vi "main.vi"() -> ()   [LabVIEW 2020, in "Resonance Curve.lvclass"]
uses:
  Resonance Curve.lvclass
  Keysight 33500B/Keysight 33511B.lvclass
  C:/Users/jhko7/Desktop/LabVIEW Programs/AFM Control/Function Generator/Function Generator.lvclass
  SR 830 & NI USB7855R/SR 830 & NI USB7855R.lvclass
  C:/Users/jhko7/Desktop/LabVIEW Programs/AFM Control/Lock-In Amplifier/Lock-In Amplifier.lvclass
  Resonance Curve Data/Resonance Curve Data.lvclass
  Resonance Curve.lvclass/Resonance Curve.ctl
panel:
  in  "Stop All":bool
  in  "Tab Control":enum32{"Measurement", "Setup"}(tab)
  in  "Stop acquisition":bool
  in  "Save Resonance Curve":bool
  out "Current amplitude":dbl
  out "Resonance curve plot":cluster{dbl[], dbl[]}[](graph)
  in  "Start Measurement":bool
  out "Current phase":dbl
  in  "error in":errorcluster
  in  "Wait time (ms)":u32=100
  in  "Driving amplitude (V rms)":dbl=0.001
  in  "Center frequency":dbl=40.0
  out "Coarse range end":dbl=32796.3
  out "Fine range end":dbl=32761.3
  out "Fine range start":dbl=32751.3
  out "Coarse range start":dbl=32716.3
  in  "Apply \nMeasurement Spec":bool
  in  "Coarse range":dbl=40.0
  in  "Fine range":dbl=5.0
  in  "Coarse increment":dbl=1.0
  in  "Fine increment":dbl=0.5
  in  "SR 830 & NI USB7855R Lock-In Amplifier":refnum<class "SR 830 & NI USB7855R.lvclass">
  in  "Keysight 33511B Waveform Generator":refnum<class "Keysight 33511B.lvclass">
  # "Measurement Frequency Select"
  # "Frequency Sweep"
  # "Resonance Curve"
  # "Range"
  # "delta"
  # "Fine"
  # "Coarse"
  # "Full Range"
  # "Fine Range"
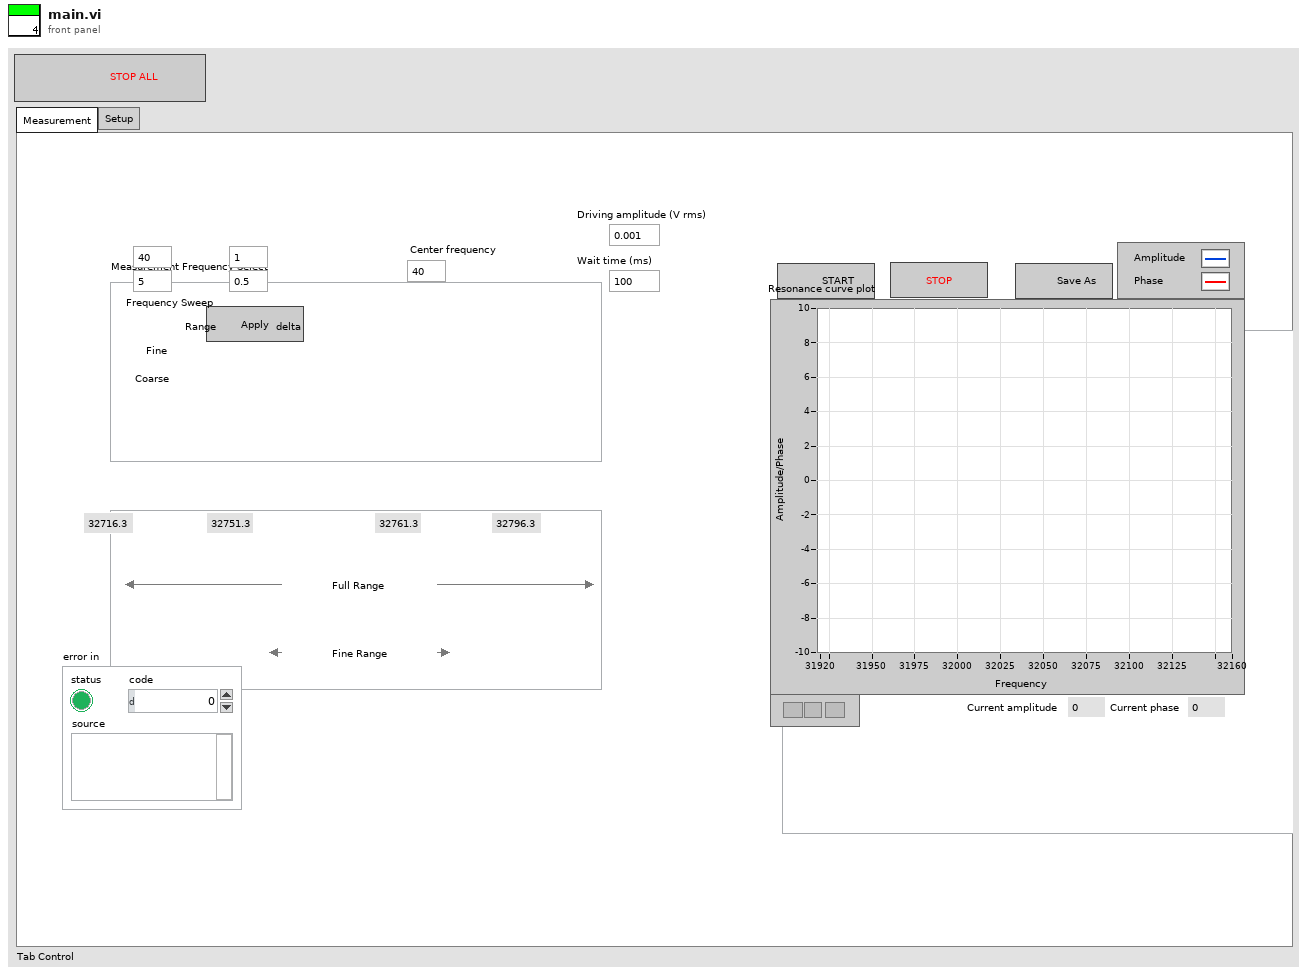
[diagram p1: front panel]
types:
  T1 = cluster{"Frequency (Hz)":dbl[], "Amplitude(V) / Phase (rad)":dbl[]}[]
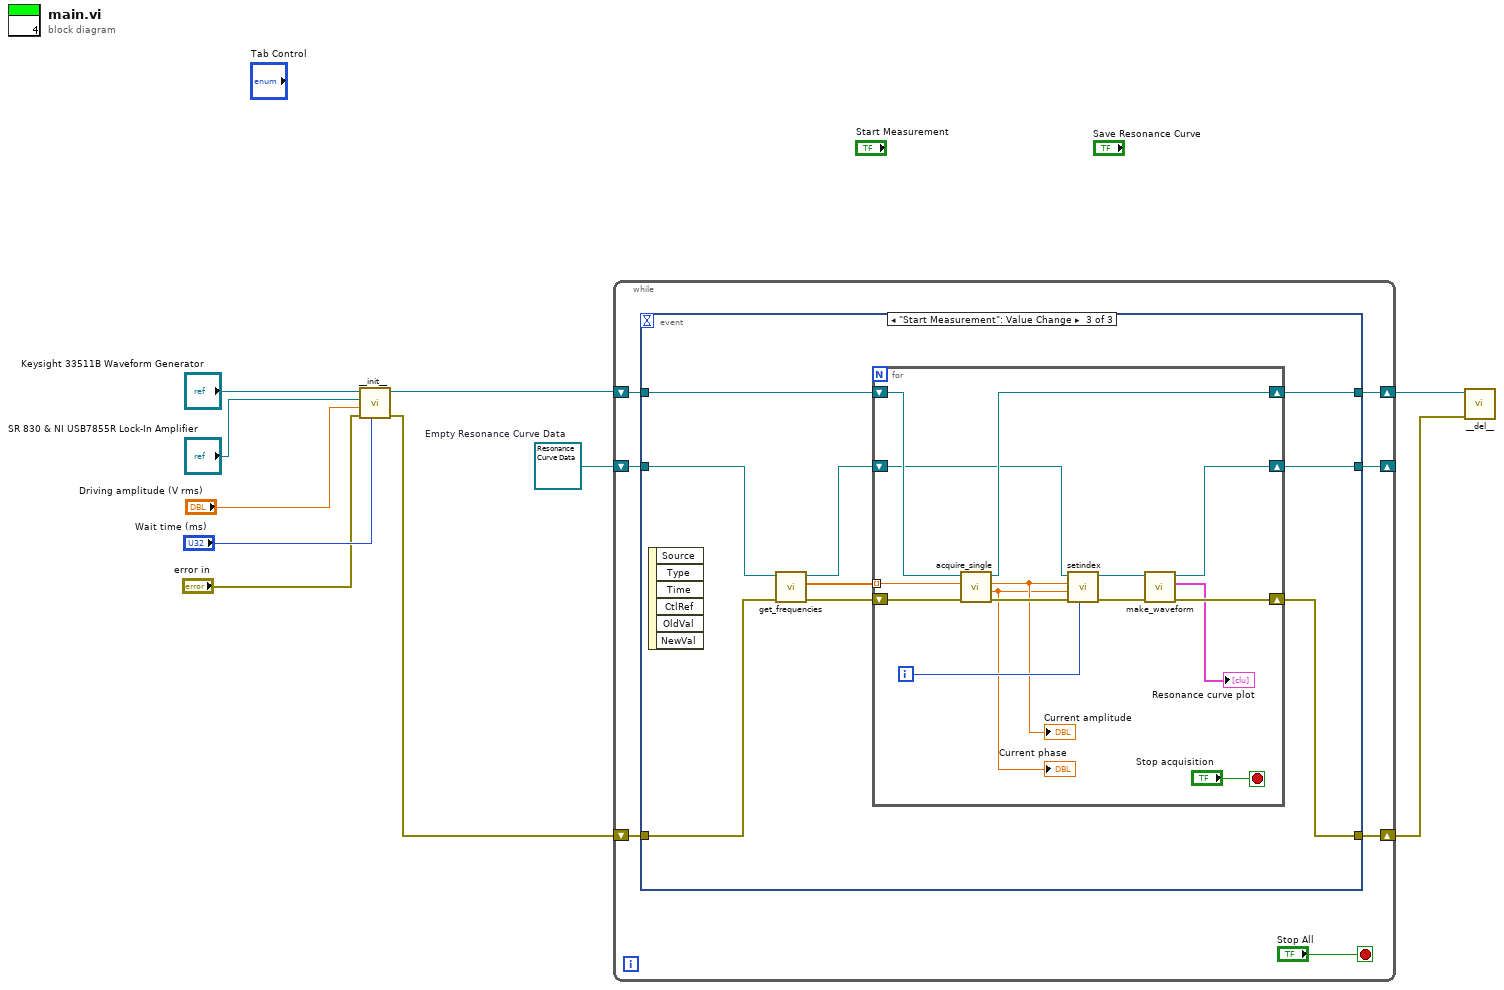
[diagram p0: block diagram]
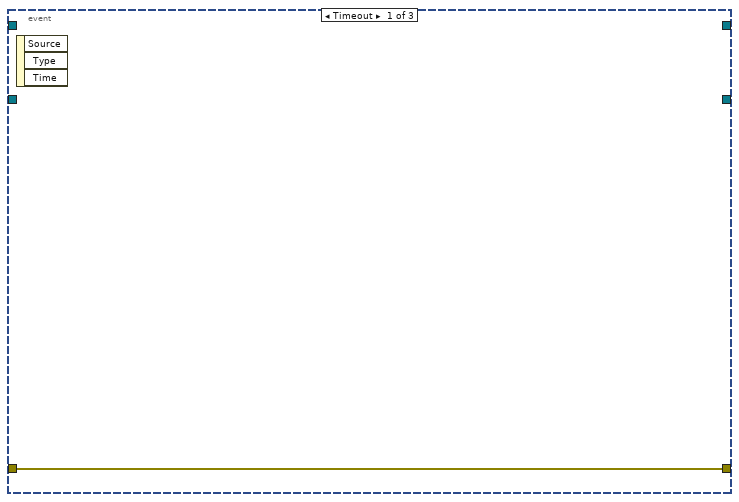
[diagram p2: hidden frame]
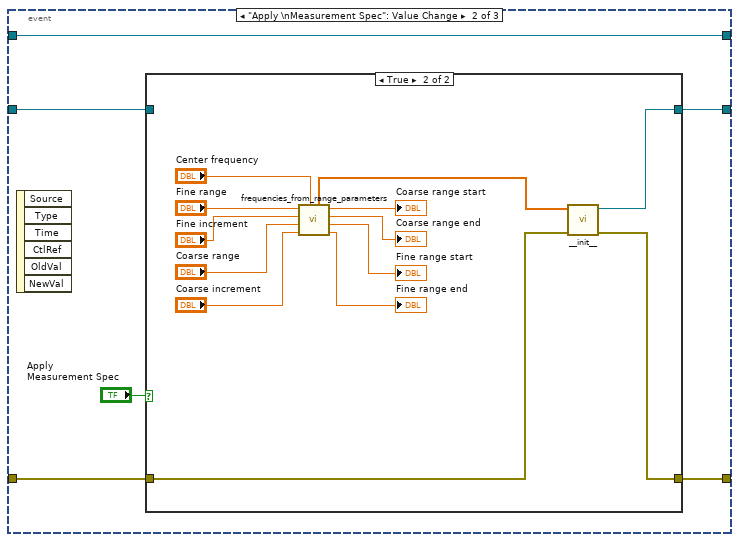
[diagram p3: hidden frame]
diagram:
  w3 = refnum<class "Resonance Curve Data.lvclass"> refnum  # Empty Resonance Curve Data
  n1 = call "__init__.vi"("Wait Time (ms)"="Wait time (ms)", "error in"="error in", "Driving Amplitude (V rms)"="Driving amplitude (V rms)", "Lock-In Amplifier"="SR 830 & NI USB7855R Lock-In Amplifier", "Function Generator"="Keysight 33511B Waveform Generator") -> ("error out"=w4:errorcluster, "Initialized Resonance Curve Measurement"=w5:refnum<class "Resonance Curve.lvclass">)  [unwired: 5 in]
  n2 = while {
    shift-right: [w14] -> w2
    shift-left: w5 -> [w17]
    shift-right: [w13] -> w1
    shift-left: w4 -> [w12]
    shift-right: [w15] -> _
    shift-left: w3 -> [w16]
    stop <- "Stop All" stop-if-true
    n3 = event shown="[2] \"Start Measurement\": Value Change" {
      selector: _ -> [_ _ _]
      dyn-events: _ -> [_ _ _]
      timeout: _ -> [_ _ _]
      tunnel: w12 -> [w18 w23 w47]
      tunnel: [w18 w22 w40] -> w13
      tunnel: w17 -> [_ w24 w42]
      tunnel: w16 -> [_ w20 w48]
      tunnel: [_ w21 w43] -> w15
      tunnel: [_ w24 w41] -> w14
      event Timeout {
        n4 = event-data() -> ()  [unwired: 1 in, 3 out]
      }
      event "Apply \nMeasurement Spec": Value Change {
        n5 = event-data() -> ()  [unwired: 1 in, 6 out]
        n6 = case shown="True" "Apply \nMeasurement Spec" {
          tunnel: w23 -> [w26 w29]
          tunnel: [w26 w28] -> w22
          tunnel: [w25 w27] -> w21
          tunnel: w20 -> [w25 _]
          frame False {
          }
          frame True {
            n7 = call "frequencies_from_range_parameters.vi"("Center frequency (Hz)"="Center frequency", "Fine increment (Hz)"="Coarse increment", "Fine range width (Hz)"="Coarse range", "Coarse increment (Hz)"="Fine increment", "Coarse range width (Hz)"="Fine range") -> ("Fine range end (Hz)"=→"Fine range end":dbl, "Fine range start (Hz)"=→"Fine range start":dbl, "Coarse range end (Hz)"=→"Coarse range end":dbl, "Coarse range start (Hz)"=→"Coarse range start":dbl, "Measurement frequencies (Hz)"=w30:dbl[])  [unwired: 2 in]
            n8 = call "__init__.vi"("error in (no error)"=w29, "Frequencies"=w30) -> ("error out"=w28:errorcluster, "Resonance Curve Data out"=w27:refnum<class "Resonance Curve Data.lvclass">)  [unwired: 8 in]
          }
        }
      }
      event "Start Measurement": Value Change {
        n9 = event-data() -> ()  [unwired: 1 in, 6 out]
        n10 = call "get_frequencies.vi"("error in"=w47, "Resonance Curve Data in"=w48) -> ("error out"=w46:errorcluster, "Frequencies (Hz)"=w45:dbl[], "Resonance Curve Data out"=w44:refnum<class "Resonance Curve Data.lvclass">)  [unwired: 7 in]
        n11 = for {
          tunnel: w45 -> [w63] mode=indexing
          shift-right: [w52] -> w43
          shift-left: w44 -> [w57]
          shift-right: [w60] -> w41
          shift-left: w42 -> [w61]
          shift-right: [w51] -> w40
          shift-left: w46 -> [w62]
          i -> [w58]
          stop <- "Stop acquisition" stop-if-true
          n12 = call-dynamic "acquire_single.vi"("error in (no error)"=w62, "Frequency (Hz)"=w63, "Resonance Curve in"=w61) -> ("error out"=w59:errorcluster, "Phase (rad)"=w55:dbl, "Amplitude (V rms)"=w56:dbl, "Resonance Curve out"=w60:refnum<class "Resonance Curve.lvclass">)  [unwired: 5 in]
          "Current amplitude" <- w56
          "Current phase" <- w55
          n13 = call "setindex.vi"("Index"=w58, "error in"=w59, "Phase (rad)"=w55, "Amplitude (V)"=w56, "Resonance Curve Data in"=w57) -> ("error out"=w53:errorcluster, "Resonance Curve Data out"=w54:refnum<class "Resonance Curve Data.lvclass">)  [unwired: 5 in]
          n14 = call "make_waveform.vi"("error in"=w53, "Resonance Curve Data in"=w54) -> ("error out"=w51:errorcluster, "2D waveform out"=→"Resonance curve plot":T1, "Resonance Curve Data out"=w52:refnum<class "Resonance Curve Data.lvclass">)  [unwired: 7 in]
        }
      }
    }
  }
  n15 = call "__del__.vi"("error in"=w1, "Resonance Curve in"=w2) -> ()  [unwired: 10 in]
